vi "BT Tx Test Fetch Results.vi"(8 "error in (no error)":errorcluster, 11 "Template Tx Test in":refnum<class "niDTS BT Tx Test.lvclass">) -> (0 "error out":errorcluster, 2 "Results":T1 {"OBW Resutls"."Stop Frequency (Hz)" format="%#_4p"; "OBW Resutls"."Start Frequency (Hz)" format="%#_4p"}, 3 "Template Tx Test out":refnum<class "niDTS BT Tx Test.lvclass">)   [LabVIEW 2015, in "niDTS BT.lvlib" / "niDTS BT Tx Test.lvclass"]
uses:
  niDTS BT Tx Test.lvclass
  Includes/niDTS BT Tx Test INC Results.ctl
  Includes/niDTS BT Tx Test INC IBE Results.ctl
  Includes/niDTS BT Tx Test INC OBW Results.ctl
  Includes/niDTS BT Tx Test INC TXP Results.ctl
  Includes/niDTS BT Tx Test INC DEVM Results.ctl
  Includes/niDTS BT Tx Test INC CF Stability Results.ctl
  Includes/niDTS BT Tx Test INC CFO Resutls.ctl
  Includes/niDTS BT Tx Test INC Character Results.ctl
  Instrument/INSTR TX/niDTS BT INSTR TX.lvclass
  Framework/Dut/Objects/BASE_class/niDTS Dut.lvclass
  niDTS BT.lvlib
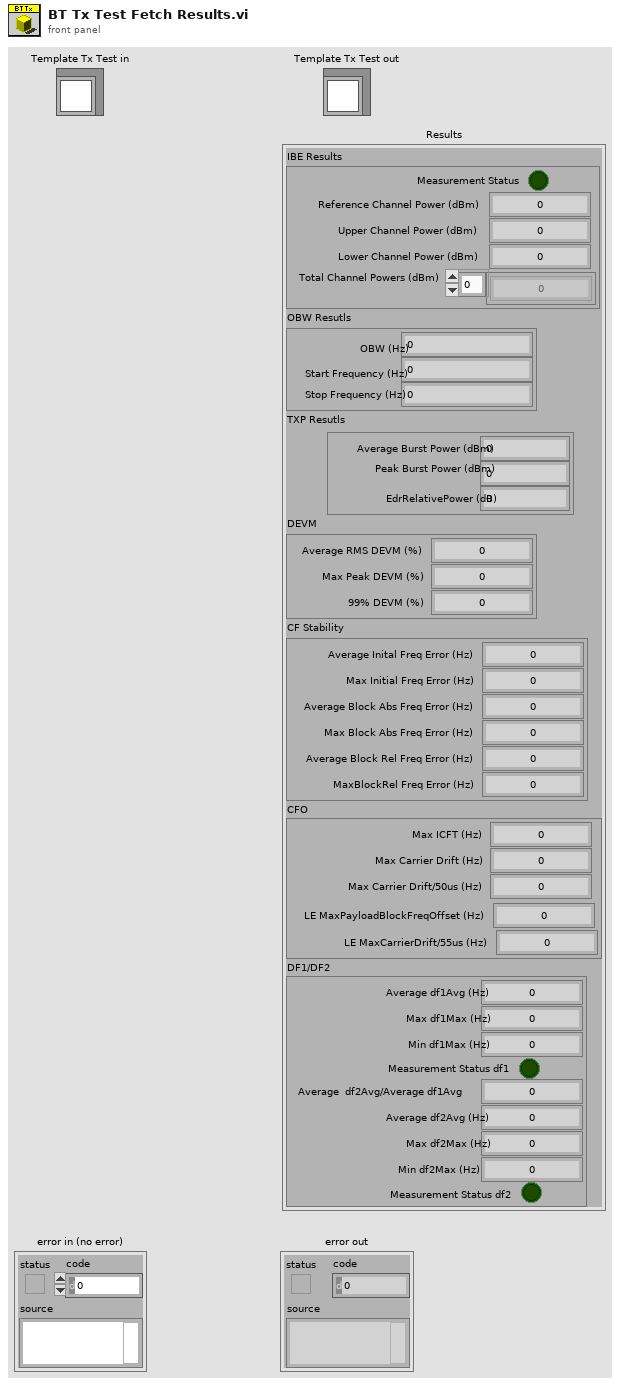
[diagram p1: front panel]
types:
  T1 = typedef "niDTS BT.lvlib/niDTS BT Tx Test INC Results.ctl" = cluster{"IBE Results":T2, "OBW Resutls":T3, "TXP Resutls":T4, "DEVM":T5, "CF Stability":T6, "CFO":T7, "DF1/DF2":T8}
  T2 = typedef "niDTS BT.lvlib/niDTS BT Tx Test INC IBE Results.ctl" = cluster{"Measurement Status":bool, "Reference Channel Power (dBm)":dbl, "Upper Channel Power (dBm)":dbl, "Lower Channel Power (dBm)":dbl, "Total Channel Powers (dBm)":dbl[]}
  T3 = typedef "niDTS BT.lvlib/niDTS BT Tx Test INC OBW Results.ctl" = cluster{"OBW (Hz)":dbl, "Start Frequency (Hz)":dbl, "Stop Frequency (Hz)":dbl}
  T4 = typedef "niDTS BT.lvlib/niDTS BT Tx Test INC TXP Results.ctl" = cluster{"Average Burst Power (dBm)":dbl, "Peak Burst Power (dBm)":dbl, "EdrRelativePower (dB)":dbl}
  T5 = typedef "niDTS BT.lvlib/niDTS BT Tx Test INC DEVM Results.ctl" = cluster{"Average RMS DEVM (%)":dbl, "Max Peak DEVM (%)":dbl, "99% DEVM (%)":dbl}
  T6 = typedef "niDTS BT.lvlib/niDTS BT Tx Test INC CF Stability Results.ctl" = cluster{"Average Inital Freq Error (Hz)":dbl, "Max Initial Freq Error (Hz)":dbl, "Average Block Abs Freq Error (Hz)":dbl, "Max Block Abs Freq Error (Hz)":dbl, "Average Block Rel Freq Error (Hz)":dbl, "MaxBlockRel Freq Error (Hz)":dbl}
  T7 = typedef "niDTS BT.lvlib/niDTS BT Tx Test INC CFO Resutls.ctl" = cluster{"Max ICFT (Hz)":dbl, "Max Carrier Drift (Hz)":dbl, "Max Carrier Drift/50us (Hz)":dbl, "LE MaxPayloadBlockFreqOffset (Hz)":dbl, "LE MaxCarrierDrift/55us (Hz)":dbl}
  T8 = typedef "niDTS BT.lvlib/niDTS BT Tx Test INC Character Results.ctl" = cluster{"Average df1Avg (Hz)":dbl, "Max df1Max (Hz)":dbl, "Min df1Max (Hz)":dbl, "Measurement Status df1":bool, "Average  df2Avg/Average df1Avg":dbl, "Average df2Avg (Hz)":dbl, "Max df2Max (Hz)":dbl, "Min df2Max (Hz)":dbl, "Measurement Status df2":bool}
  T9 = typedef "niDTS Framework.lvlib/niDTS Dut INC Handle.ctl" = refnum<data-value>
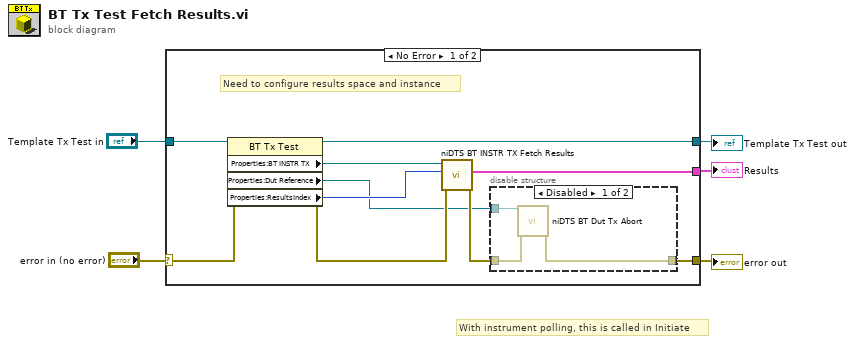
[diagram p0: block diagram]
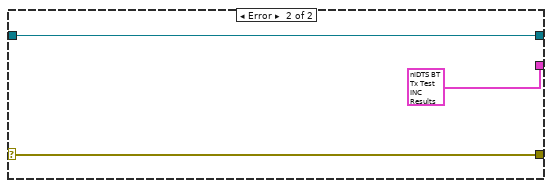
[diagram p3: hidden frame]
diagram:
  # "With instrument polling, this is called in Initiate"
  n1 = case shown="No Error" "error in (no error)" {
    selector: "error in (no error)" -> [w12 w22]
    tunnel: [w9 w22] -> w4
    tunnel: [w15 w21] -> w2
    tunnel: "Template Tx Test in" -> [w6 w21]
    tunnel: [w13 T1 {"IBE Results"={"Measurement Status"=FALSE, "Reference Channel Power (dBm)"=0.0, "Upper Channel Power (dBm)"=0.0, "Lower Channel Power (dBm)"=0.0, "Total Channel Powers (dBm)"=[]}, "OBW Resutls"={"OBW (Hz)"=0.0, "Start Frequency (Hz)"=0.0, "Stop Frequency (Hz)"=0.0}, "TXP Resutls"={"Average Burst Power (dBm)"=0.0, "Peak Burst Power (dBm)"=0.0, "EdrRelativePower (dB)"=0.0}, "DEVM"={"Average RMS DEVM (%)"=0.0, "Max Peak DEVM (%)"=0.0, "99% DEVM (%)"=0.0}, "CF Stability"={"Average Inital Freq Error (Hz)"=0.0, "Max Initial Freq Error (Hz)"=0.0, "Average Block Abs Freq Error (Hz)"=0.0, "Max Block Abs Freq Error (Hz)"=0.0, "Average Block Rel Freq Error (Hz)"=0.0, "MaxBlockRel Freq Error (Hz)"=0.0}, "CFO"={"Max ICFT (Hz)"=0.0, "Max Carrier Drift (Hz)"=0.0, "Max Carrier Drift/50us (Hz)"=0.0, "LE MaxPayloadBlockFreqOffset (Hz)"=0.0, "LE MaxCarrierDrift/55us (Hz)"=0.0}, "DF1/DF2"={"Average df1Avg (Hz)"=0.0, "Max df1Max (Hz)"=0.0, "Min df1Max (Hz)"=0.0, "Measurement Status df1"=FALSE, "Average  df2Avg/Average df1Avg"=0.0, "Average df2Avg (Hz)"=0.0, "Max df2Max (Hz)"=0.0, "Min df2Max (Hz)"=0.0, "Measurement Status df2"=FALSE}} ("Results")] -> w1
    frame No Error {
      # "Need to configure results space and instance"
      n2 = property class="BT Tx Test"(reference=w6, error in=w12) -> (reference out=w15:refnum<class "niDTS BT Tx Test.lvclass">, error out=w11:errorcluster, "Properties:BT INSTR TX"=w14:refnum<class "niDTS BT INSTR TX.lvclass">, "Properties:Dut Reference"=w7:T9, "Properties:ResultsIndex"=w8:u8)
      n3 = call-dynamic "niDTS BT INSTR TX Fetch Results.vi"("error in (no error)"=w11, "ResultsIndex"=w8, "niDTS BT INSTR TX in"=w14) -> ("error out"=w10:errorcluster, "Results"=w13:T1)  [unwired: 6 in, 1 out]
      n4 = disable-structure shown="Disabled" {
        disable-tunnel: w10 -> [w18 w19]
        disable-tunnel: [w17 w19] -> w9
        disable-tunnel: w7 -> [w16 _]
        frame Disabled {
          n5 = call "niDTS BT Dut Tx Abort.vi"("BT Dut Handle in"=w16, "error in (no error)"=w18) -> ("error out"=w17:errorcluster)  [unwired: 12 in, 1 out]
        }
        frame Enabled {
        }
      }
    }
    frame Error {
    }
  }
  "error out" <- w4
  "Template Tx Test out" <- w2
  "Results" <- w1
